vi "RunMeas.vi"(8 "error in (no error)":errorcluster, 11 "PacificPowerSource in":refnum<class "PacificPowerSource.lvclass">) -> (0 "error out":errorcluster, 2 "variant":variant, 3 "PacificPowerSource out":refnum<class "PacificPowerSource.lvclass">)   [LabVIEW 2018, in "AcPwrPlugins.lvlib" / "PacificPowerSource.lvclass"]
doc: "This VI (may) start and retrieve measurements from the instruments."
uses:
  PacificPowerSource.lvclass
  AcPwrShared/clMeasurmentData.ctl
  AcPwrShared/clAcPwrAttributes.ctl
  AcPwrShared/AcPwrShared.lvlib
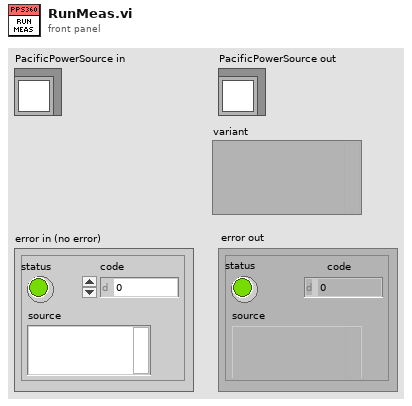
[diagram p1: front panel]
types:
  T1 = typedef "AcPwrPlugins.lvlib/PacificPowerSource.lvclass/Device(s)Settings.ctl" = cluster{"MeasName":string, "Modules":cluster{"Handle":string, "Connected":bool, "Clear Device (F)":bool, "btnIdQuery":bool, "btnReset":bool, "Program #":cluster{"Phase B (Degrees)":i32, "Waveform A (1: Sine)":i32, "Voltage Level (Va)":dbl, "Program Number (0)":i32, "Voltage Level (Vb) ":dbl, "Form (3: Three)":u16, "Coupling  (0: Direct)":u16, "Frequency (45Hz)":dbl, "Current Limit (40A)":dbl, "Phase C (Degrees)":i32, "Voltage Level (Vc)":dbl, "Waveform B (1: Sine)":i32, "Waveform C (1: Sine)":i32}[], "Impedance Parameters (off, 0.00)":cluster{"State":bool, "Impedance":dbl}, "Transient Execution (F)":bool, "OutputEnabled":bool, "Source Range":cluster{"Frequency Minimum (45 Hz)":dbl, "Frequency Maximum (1200 Hz)":dbl, "Voltage Maximum (V)":dbl, "Voltage Minimum (V)":dbl, "Range Control (0: Auto)":u16, "Initial Voltage (0V)":dbl, "Frequency Range (600Hz)":u16}, "Port Type":enum16{"GPIB", "Serial"}}[]}
  T2 = typedef "AcPwrPlugins.lvlib/PacificPowerSource.lvclass/Measurements.ctl" = cluster{"Handle":string, "Name":string, "Enabled ":bool, "Measurement Value":dbl, "Channel Name":enum16{"A", "B", "C"}, "Measurement Type ":T3}[]
  T3 = typedef "AcPwrPlugins.lvlib/PacificPowerSource.lvclass/MeasurementType.ctl" = enum16{"Voltage RMS L-N", "Voltage RMS L-L", "Frequency", "Current RMS", "Current Peak", "Crest Factor", "Power Factor", "Power VA", "Real Power"}
  T4 = typedef "AcPwrShared.lvlib/clMeasurmentData.ctl" = cluster{"MeasName":string, "XML Data":string, "WaveformData":waveform(dbl)[]}
  T5 = typedef "AcPwrShared.lvlib/clAcPwrAttributes.ctl" = cluster{"ProtectionStatusString":string, "Handle_MeasurementType":string, "Status Byte Register":cluster{"Busy":bool, "Remote Mode":bool, "Error in Queue":bool, "QUES=Questionable Status Summary":bool, "MAV = Message Available":bool, "ESB = Event Status Byte Summary":bool, "RQS = Request for Service":bool, "OPER = Operation Event Summary":bool}}
  T6 = cluster{"Vrms A":dbl, "Vrms B":dbl, "Vrms C":dbl, "Vrms A-B":dbl, "Vrms B-C":dbl, "Vrms C-A":dbl, "Irms A":dbl, "Irms B":dbl, "Irms C":dbl, "Ipeak A":dbl, "Ipeak B":dbl, "Ipeak C":dbl, "Icrest A":dbl, "Icrest B":dbl, "Icrest C":dbl, "KW   A":dbl, "KW   B":dbl, "KW   C":dbl, "KVA   A":dbl, "KVA   B":dbl, "KVA   C":dbl, "PF   A":dbl, "PF   B":dbl, "PF   C":dbl, "Frequency":dbl}
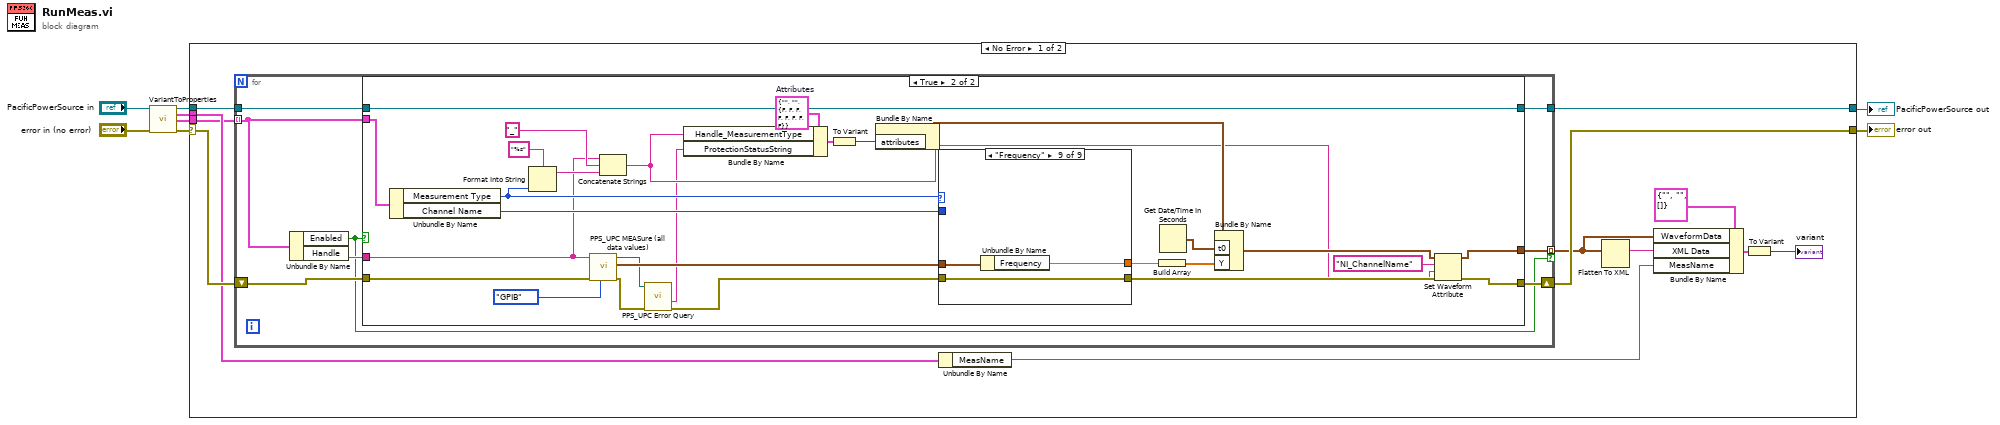
[diagram p0: block diagram]
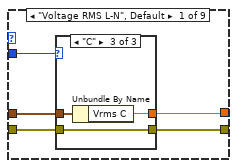
[diagram p3: hidden frame]
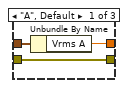
[diagram p4: hidden frame]
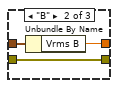
[diagram p5: hidden frame]
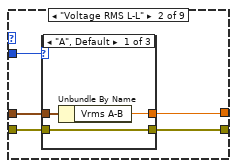
[diagram p6: hidden frame]
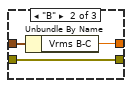
[diagram p7: hidden frame]
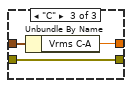
[diagram p8: hidden frame]
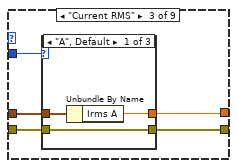
[diagram p9: hidden frame]
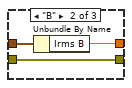
[diagram p10: hidden frame]
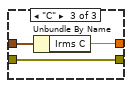
[diagram p11: hidden frame]
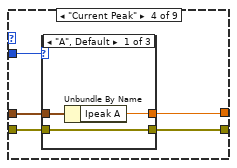
[diagram p12: hidden frame]
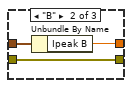
[diagram p13: hidden frame]
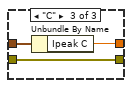
[diagram p14: hidden frame]
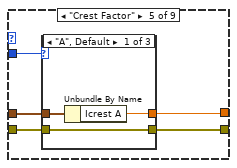
[diagram p15: hidden frame]
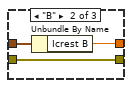
[diagram p16: hidden frame]
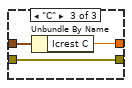
[diagram p17: hidden frame]
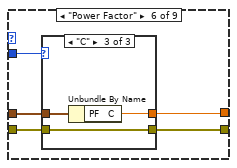
[diagram p18: hidden frame]
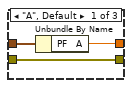
[diagram p19: hidden frame]
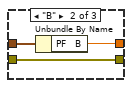
[diagram p20: hidden frame]
diagram:
  n1 = call "VariantToProperties.vi"("PacificPowerSource in"="PacificPowerSource in", "error in (no error)"="error in (no error)") -> ("PacificPowerSource out"=w5:refnum<class "PacificPowerSource.lvclass">, "Device(s)Settings"=w2:T1, "Measurements"=w1:T2, "error out"=w3:errorcluster)  [unwired: 7 in, 3 out]
  n2 = case shown="No Error" w3 {
    selector: w3 -> [w19 w178]
    tunnel: [w15 w178] -> w7
    tunnel: [w18 w179] -> w8
    tunnel: w5 -> [w20 w179]
    tunnel: w2 -> [w17 _]
    tunnel: w1 -> [w16 _]
    frame No Error {
      n3 = for {
        tunnel: w16 -> [w28] mode=indexing
        tunnel: [w27] -> w9 mode=indexing if=w21
        shift-right: [w24] -> w15
        shift-left: w19 -> [w25]
        tunnel: w20 -> [w23]
        tunnel: [w22] -> w18
        n4 = Unbundle By Name(w28) -> ("Enabled"=w21:bool, "Handle"=w26:string)
        n5 = case shown="True" w21 {
          tunnel: w28 -> [_ w53]
          tunnel: [_ w37] -> w27
          tunnel: w25 -> [w30 w57]
          tunnel: w26 -> [_ w42]
          tunnel: [w30 w38] -> w24
          tunnel: w23 -> [w29 w54]
          tunnel: [w29 w54] -> w22
          frame False {
          }
          frame True {
            w45 = T5 {"ProtectionStatusString"="", "Handle_MeasurementType"="", "Status Byte Register"={"Busy"=FALSE, "Remote Mode"=FALSE, "Error in Queue"=FALSE, "QUES=Questionable Status Summary"=FALSE, "MAV = Message Available"=FALSE, "ESB = Event Status Byte Summary"=FALSE, "RQS = Request for Service"=FALSE, "OPER = Operation Event Summary"=FALSE}}  # Attributes
            n6 = Unbundle By Name(w53) -> ("Measurement Type"=w43:T3, "Channel Name"=w55:enum16{"A", "B", "C"})
            n7 = Format Into String(format string="%s", w43) -> (resulting string=w46:string)  [unwired: 2 in, 1 out]
            n8 = call <instrlib>:"PPS_UPC MEASure (all data values).vi"("Port Type"=enum16{"GPIB", "Serial"}."GPIB", "error in (no error)"=w57, "VISA session"=w42) -> ("error out"=w33:errorcluster, "Metered Data"=w56:T6, "dup VISA session"=w34:refnum<visa-resource-name>)  [unwired: 5 in, 1 out]
            n9 = Concatenate Strings(w42, "_", w46) -> (w35:string)
            n10 = call <instrlib>:"PPS_UPC Error Query.vi"("error in (no error)"=w33, "VISA session"=w34) -> ("error out"=w32:errorcluster, "Error Message"=w31:string)  [unwired: 6 in, 2 out]
            n11 = Bundle By Name(cluster=w45, "Handle_MeasurementType"=w35, "ProtectionStatusString"=w31) -> (w44:T5)
            n12 = To Variant(anything=w44) -> (Variant=w48:variant)
            n13 = Bundle By Name("attributes"=w48) -> (w41:waveform(dbl))  [unwired: 1 in]
            n14 = case shown="\"Frequency\"" w43 {
              tunnel: w56 -> [w60 w74 w88 w102 w116 w130 w146 w162 w176]
              tunnel: [w59 w73 w87 w101 w115 w129 w144 w160 w175] -> w50
              tunnel: w32 -> [w63 w77 w91 w105 w119 w133 w149 w165 w177]
              tunnel: [w62 w76 w90 w104 w118 w132 w148 w164 w177] -> w39
              tunnel: w55 -> [w61 w75 w89 w103 w117 w131 w147 w163 _]
              frame "Voltage RMS L-N", Default {
                n15 = case shown="\"C\"" w61 {
                  tunnel: w63 -> [w66 w69 w72]
                  tunnel: [w66 w69 w72] -> w62
                  tunnel: w60 -> [w65 w68 w71]
                  tunnel: [w64 w67 w70] -> w59
                  frame "A", Default {
                    n16 = Unbundle By Name(w65) -> ("Vrms A"=w64:dbl)
                  }
                  frame "B" {
                    n17 = Unbundle By Name(w68) -> ("Vrms B"=w67:dbl)
                  }
                  frame "C" {
                    n18 = Unbundle By Name(w71) -> ("Vrms C"=w70:dbl)
                  }
                }
              }
              frame "Voltage RMS L-L" {
                n19 = case shown="\"A\", Default" w75 {
                  tunnel: w77 -> [w80 w83 w86]
                  tunnel: [w80 w83 w86] -> w76
                  tunnel: w74 -> [w79 w82 w85]
                  tunnel: [w78 w81 w84] -> w73
                  frame "A", Default {
                    n20 = Unbundle By Name(w79) -> ("Vrms A-B"=w78:dbl)
                  }
                  frame "B" {
                    n21 = Unbundle By Name(w82) -> ("Vrms B-C"=w81:dbl)
                  }
                  frame "C" {
                    n22 = Unbundle By Name(w85) -> ("Vrms C-A"=w84:dbl)
                  }
                }
              }
              frame "Current RMS" {
                n23 = case shown="\"A\", Default" w89 {
                  tunnel: w91 -> [w94 w97 w100]
                  tunnel: [w94 w97 w100] -> w90
                  tunnel: w88 -> [w93 w96 w99]
                  tunnel: [w92 w95 w98] -> w87
                  frame "A", Default {
                    n24 = Unbundle By Name(w93) -> ("Irms A"=w92:dbl)
                  }
                  frame "B" {
                    n25 = Unbundle By Name(w96) -> ("Irms B"=w95:dbl)
                  }
                  frame "C" {
                    n26 = Unbundle By Name(w99) -> ("Irms C"=w98:dbl)
                  }
                }
              }
              frame "Current Peak" {
                n27 = case shown="\"A\", Default" w103 {
                  tunnel: w105 -> [w108 w111 w114]
                  tunnel: [w108 w111 w114] -> w104
                  tunnel: w102 -> [w107 w110 w113]
                  tunnel: [w106 w109 w112] -> w101
                  frame "A", Default {
                    n28 = Unbundle By Name(w107) -> ("Ipeak A"=w106:dbl)
                  }
                  frame "B" {
                    n29 = Unbundle By Name(w110) -> ("Ipeak B"=w109:dbl)
                  }
                  frame "C" {
                    n30 = Unbundle By Name(w113) -> ("Ipeak C"=w112:dbl)
                  }
                }
              }
              frame "Crest Factor" {
                n31 = case shown="\"A\", Default" w117 {
                  tunnel: w119 -> [w122 w125 w128]
                  tunnel: [w122 w125 w128] -> w118
                  tunnel: w116 -> [w121 w124 w127]
                  tunnel: [w120 w123 w126] -> w115
                  frame "A", Default {
                    n32 = Unbundle By Name(w121) -> ("Icrest A"=w120:dbl)
                  }
                  frame "B" {
                    n33 = Unbundle By Name(w124) -> ("Icrest B"=w123:dbl)
                  }
                  frame "C" {
                    n34 = Unbundle By Name(w127) -> ("Icrest C"=w126:dbl)
                  }
                }
              }
              frame "Power Factor" {
                n35 = case shown="\"C\"" w131 {
                  tunnel: w133 -> [w136 w139 w142]
                  tunnel: [w136 w139 w142] -> w132
                  tunnel: w130 -> [w135 w138 w141]
                  tunnel: [w134 w137 w140] -> w129
                  frame "A", Default {
                    n36 = Unbundle By Name(w135) -> ("PF   A"=w134:dbl)
                  }
                  frame "B" {
                    n37 = Unbundle By Name(w138) -> ("PF   B"=w137:dbl)
                  }
                  frame "C" {
                    n38 = Unbundle By Name(w141) -> ("PF   C"=w140:dbl)
                  }
                }
              }
              frame "Power VA" {
                n39 = case shown="\"A\", Default" w147 {
                  tunnel: w149 -> [w152 w155 w158]
                  tunnel: [w152 w155 w158] -> w148
                  tunnel: w146 -> [w151 w154 w157]
                  tunnel: [w150 w153 w156] -> w145
                  frame "A", Default {
                    n40 = Unbundle By Name(w151) -> ("KVA   A"=w150:dbl)
                  }
                  frame "B" {
                    n41 = Unbundle By Name(w154) -> ("KVA   B"=w153:dbl)
                  }
                  frame "C" {
                    n42 = Unbundle By Name(w157) -> ("KVA   C"=w156:dbl)
                  }
                }
                n43 = Multiply(x=1000.0, y=w145) -> (x*y=w144:dbl)
              }
              frame "Real Power" {
                n44 = case shown="\"C\"" w163 {
                  tunnel: w165 -> [w168 w171 w174]
                  tunnel: [w168 w171 w174] -> w164
                  tunnel: w162 -> [w167 w170 w173]
                  tunnel: [w166 w169 w172] -> w161
                  frame "A", Default {
                    n45 = Unbundle By Name(w167) -> ("KW   A"=w166:dbl)
                  }
                  frame "B" {
                    n46 = Unbundle By Name(w170) -> ("KW   B"=w169:dbl)
                  }
                  frame "C" {
                    n47 = Unbundle By Name(w173) -> ("KW   C"=w172:dbl)
                  }
                }
                n48 = Multiply(x=1000.0, y=w161) -> (x*y=w160:dbl)
              }
              frame "Frequency" {
                n49 = Unbundle By Name(w176) -> ("Frequency"=w175:dbl)
              }
            }
            n50 = Build Array(w50) -> (w52:dbl[])
            n51 = Get Date/Time In Seconds() -> (seconds since 1Jan1904=w51:timestamp)
            n52 = Bundle By Name(cluster=w41, "t0"=w51, "Y"=w52) -> (w36:waveform(dbl))
            n53 = Set Waveform Attribute(4:w39, 5:w35, 6:"NI_ChannelName" ("name"), 7:w36) -> (0:w38:errorcluster, 3:w37:waveform(dbl))  [unwired: 1 out]
          }
        }
      }
      n54 = Unbundle By Name(w17) -> ("MeasName"=w10:string)
      n55 = Flatten To XML(anything=w9) -> (xml string=w12:string)
      n56 = Bundle By Name(cluster=T4 {"MeasName"="", "XML Data"="", "WaveformData"=[]} ("MeasurmentDataCluster"), "WaveformData"=w9, "XML Data"=w12, "MeasName"=w10) -> (w13:T4)
      n57 = To Variant(anything=w13) -> (Variant=→"variant":variant)
    }
    frame Error {
    }
  }
  "PacificPowerSource out" <- w8
  "error out" <- w7
